vi "Get Child 1 level under Root Item.vi"(11 "TreeControl in":refnum<vi>) -> (2 "All Child under Root":string[](array[string]), 3 "TreeControl out":refnum<vi>)   [LabVIEW 2021]
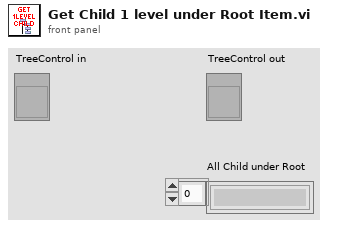
[diagram p1: front panel]
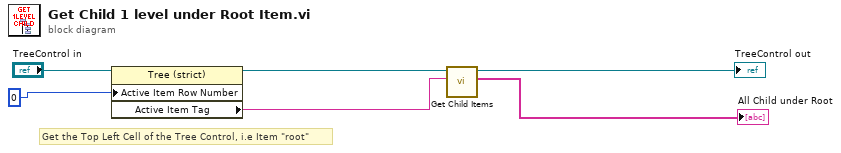
[diagram p0: block diagram]
diagram:
  # "Get the Top Left Cell of the Tree Control, i.e Item \"root\""
  n1 = property on="Property Node" class="Tree (strict)"(reference="TreeControl in", "Active Item Row Number"=0 ("Active Item:Row Number")) -> (reference out=w5:refnum<vi>, "Active Item Tag"=w1:string)  [unwired: 1 in, 1 out]
  n2 = call "Get Child Items.vi"("Node"=w1, "TreeControl in"=w5) -> ("Child Array"=→"All Child under Root":string[], "TreeControl out"=→"TreeControl out":refnum<vi>)  [unwired: 8 in]
